vi "Advanced settings MAX.vi"(1 "Admin Path":string="C:\\Data Log\\Admin") -> (0 "output cluster":T1)   [LabVIEW 2014]
uses:
  <vilib>/Utility/file.llb/Read From Spreadsheet File (DBL).vi
panel:
  out "SMS Recipients":u32
  in  "SMS":bool
  in  "Mexa 7170":bool
  out "Boolean":bool
  in  "Leak Test":bool
  in  "OK Button":bool
  in  "Bottle":bool
  in  "Logging":bool
  in  "System":bool
  in  "Lambda":bool
  out "Tab Control":T2(tab)
  in  "Inlet TC":dbl=1.0 min=1.0 max=32.0
  in  "Bed TC":dbl=1.0 min=1.0 max=32.0
  in  "Cycle Length":dbl=500.0
  in  "Heat Load Control":bool
  in  "Purge Duration":dbl=30.0
  in  "Reference Temp":dbl=700.0
  in  "Target Heat Load":dbl
  in  "C Factor":dbl=21000.0
  in  "Directory":string="C:\\Data Log"
  in  "ETAS":bool
  in  "MKS":bool
  in  "Mexa 1":bool
  in  "Mexa 2":bool
  in  "Mexa 3":bool
  in  "Log Interval":dbl=4.0
  in  "Vehicle Name":string="V1"
  in  "Nicky":bool
  in  "Kurtis":bool
  in  "Andy":bool
  in  "Ryan":bool
  in  "Liam":bool
  in  "Matthew":bool
  in  "Calvin":bool
  in  "Text Alerts":bool
  in  "Lambda Control On/Off":bool
  in  "D":dbl min=0.0 max=100.0
  in  "I":dbl min=0.0 max=100.0
  in  "P":dbl min=0.0 max=100.0
  in  "Lambda Target":dbl min=0.0 max=100.0
  in  "O2 Concentration":dbl=100.0 min=0.0 max=100.0
  in  "Propane":bool
  in  "CO Concentration":dbl=100.0 min=0.0 max=100.0
  in  "HC Concentration":dbl=100.0 min=0.0 max=100.0
  in  "NOx Concentration":dbl=100.0 min=0.0 max=100.0
  in  "Air Bal":bool
  in  "N2":bool
  in  "Duration Leak Test":dbl min=0.0 max=100.0
  # "Advanced Settings"
  # "System Settings"
  # "s"
  # "hr"
  # "Advanced Settings"
  # "Data Log Settings"
  # "hr"
  # "Advanced Settings"
  # "SMS Alert Settings"
  # "SMS Recipients"
  # "Advanced Settings"
  # "Lambda Control Settings"
  # "Advanced Settings"
  # "Gas Settings"
  # "%"
  # "%"
  # "%"
  # "%"
  # "Advanced Settings"
  # "Leak Test Settings"
  # "s"
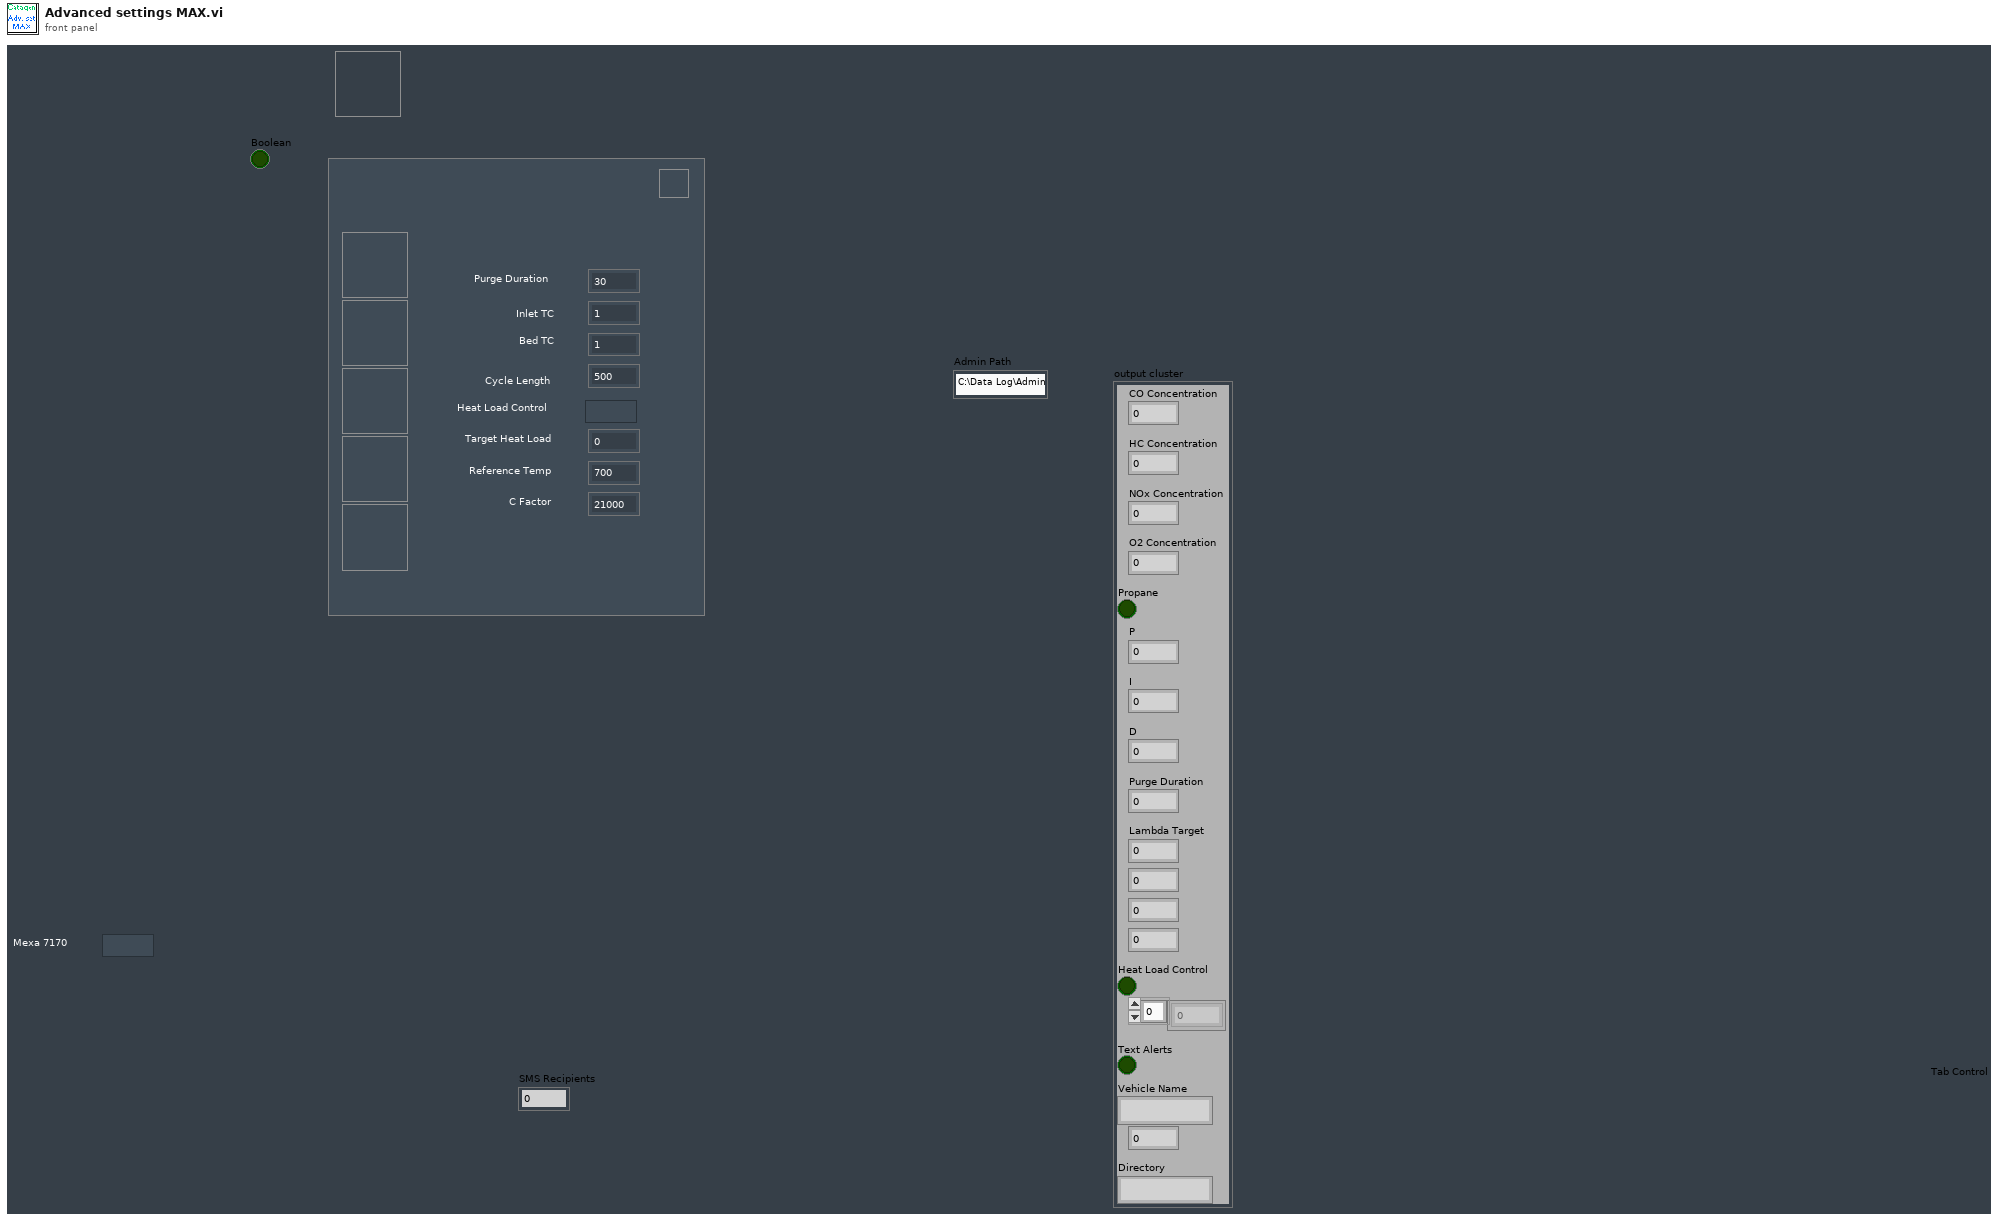
[diagram p1: front panel]
types:
  T1 = cluster{"CO Concentration":dbl, "HC Concentration":dbl, "NOx Concentration":dbl, "O2 Concentration":dbl, "Propane":bool, "P":dbl, "I":dbl, "D":dbl, "Purge Duration":dbl, "Lambda Target":dbl, dbl, u32, dbl, "Heat Load Control":bool, dbl[], "Text Alerts":bool, "Vehicle Name":string, u32, "Directory":string}
  T2 = enum32{"System ", "Logging", "SMS", "Lambda", "Bottle", "Leak Test"}
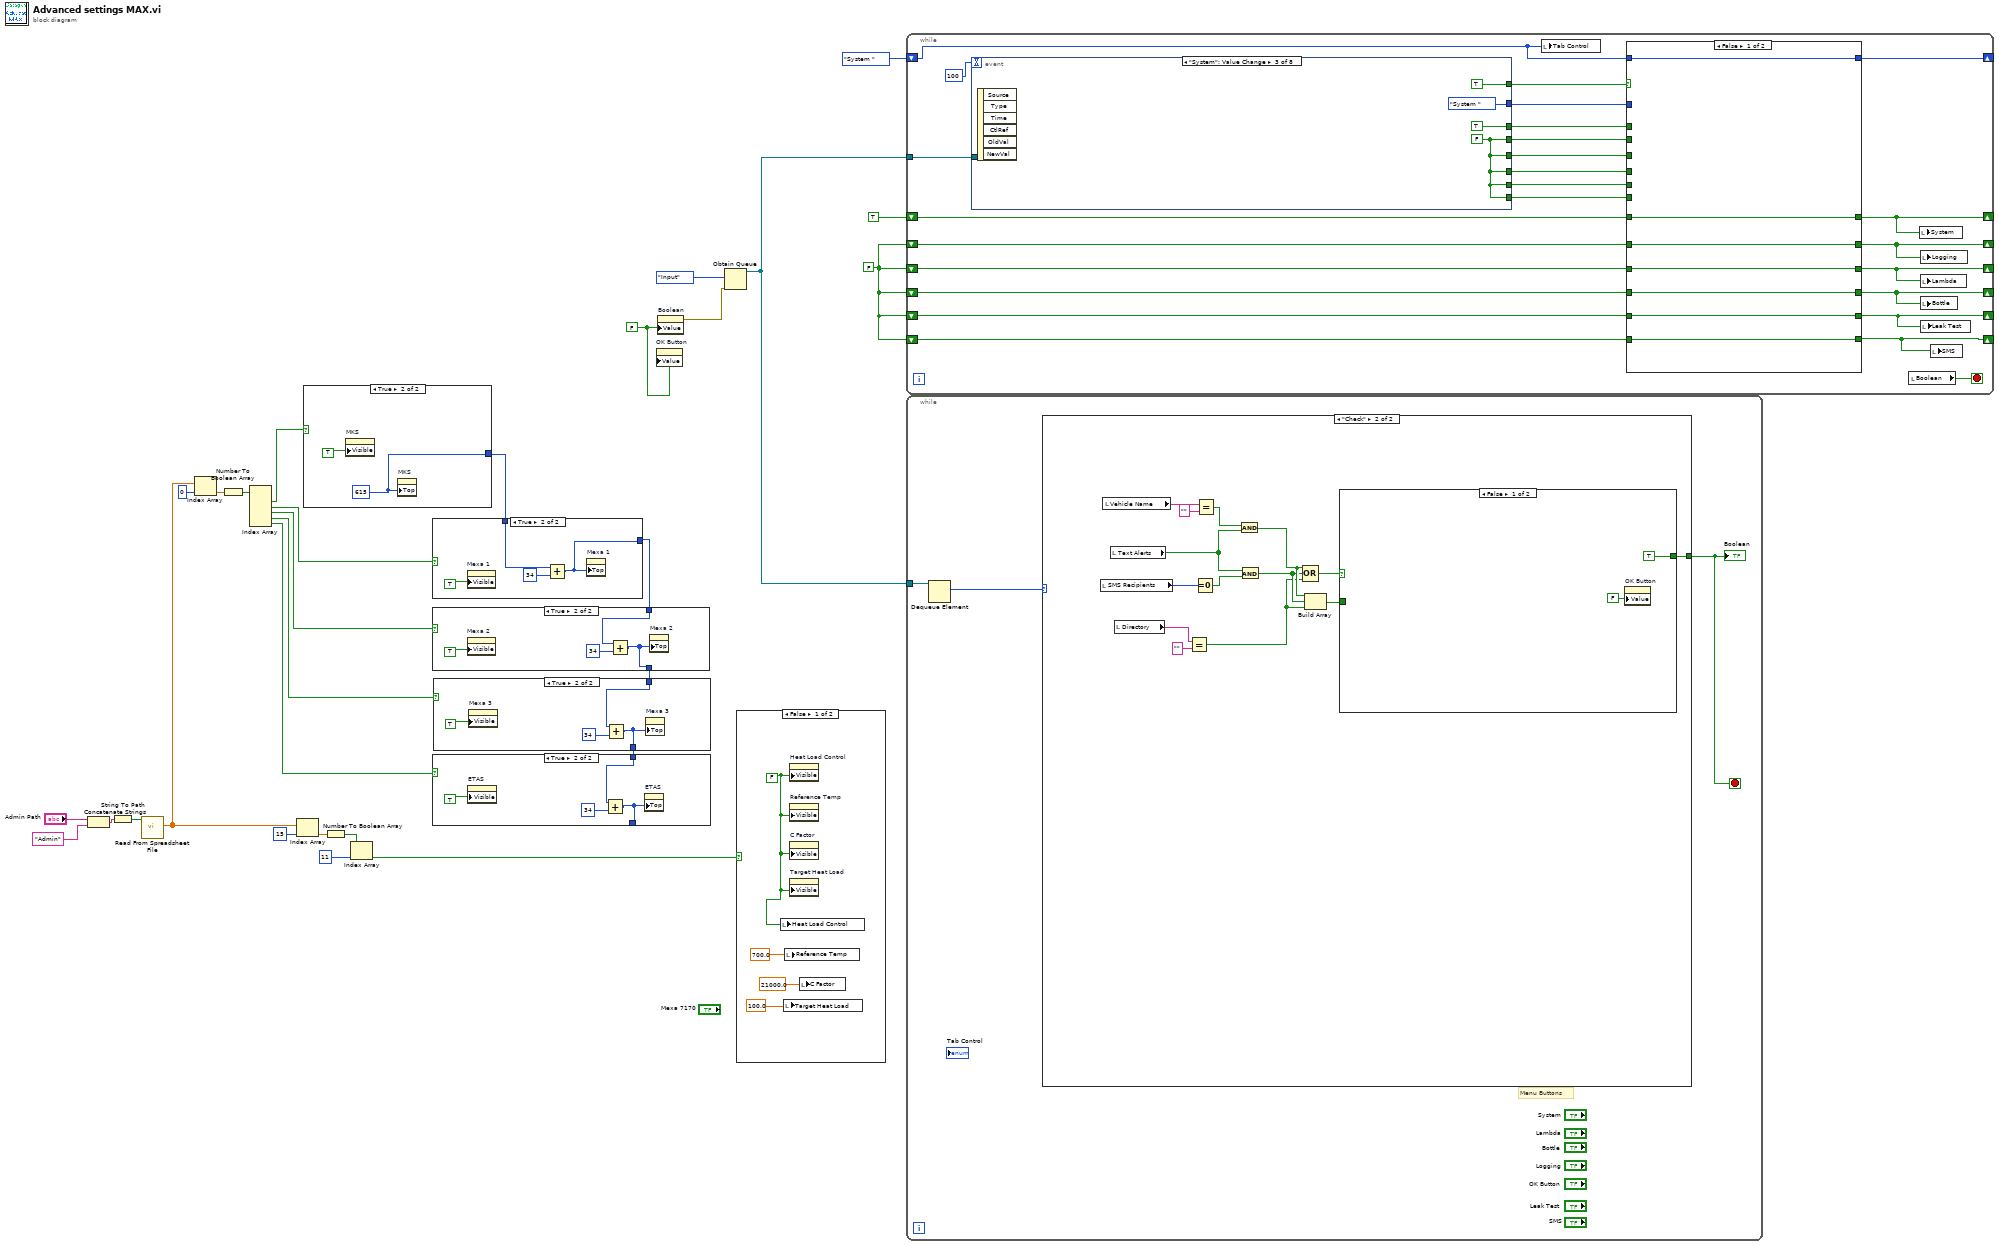
[diagram p0: block diagram]
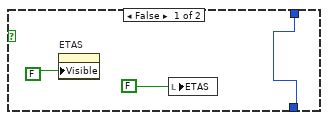
[diagram p2: hidden frame]
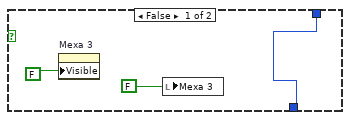
[diagram p3: hidden frame]
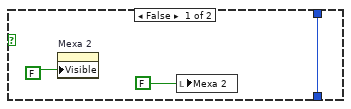
[diagram p4: hidden frame]
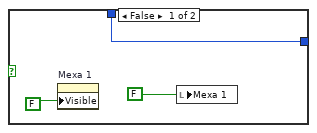
[diagram p5: hidden frame]
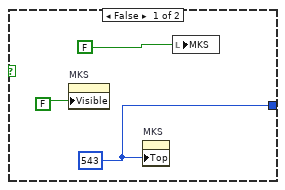
[diagram p6: hidden frame]
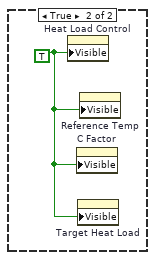
[diagram p7: hidden frame]
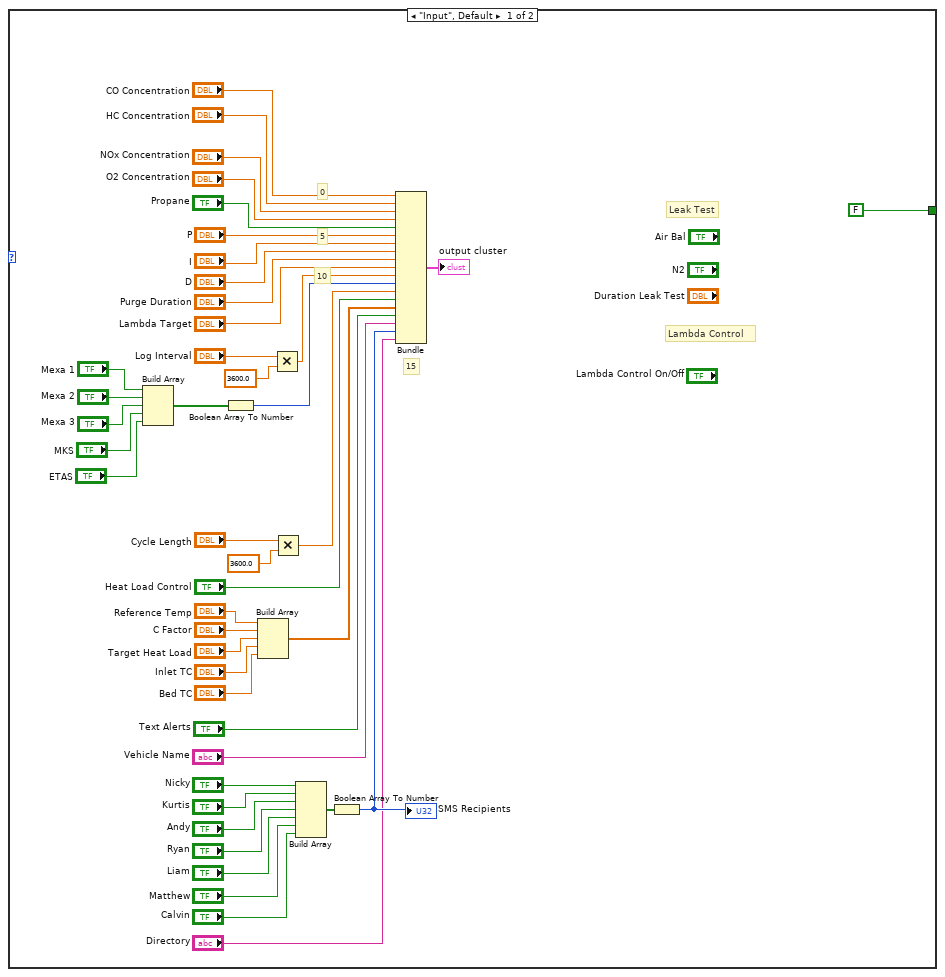
[diagram p8: hidden frame]
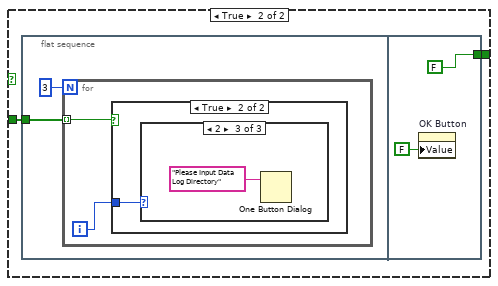
[diagram p9: hidden frame]
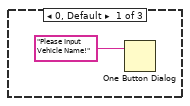
[diagram p11: hidden frame]
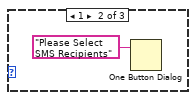
[diagram p12: hidden frame]
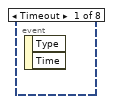
[diagram p14: hidden frame]
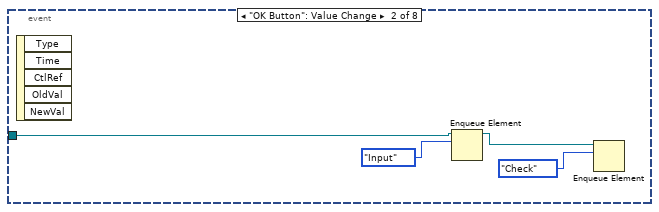
[diagram p15: hidden frame]
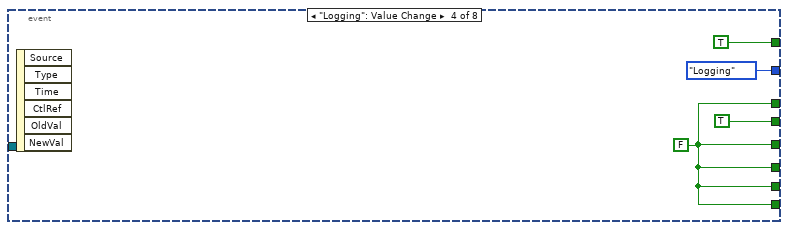
[diagram p16: hidden frame]
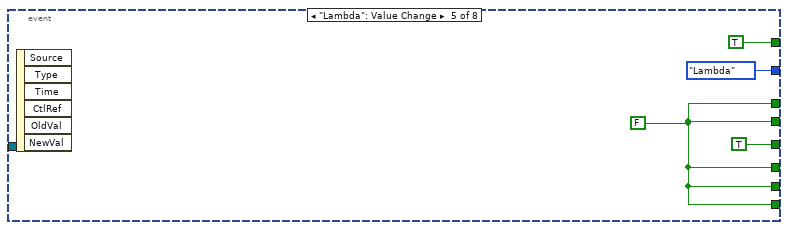
[diagram p17: hidden frame]
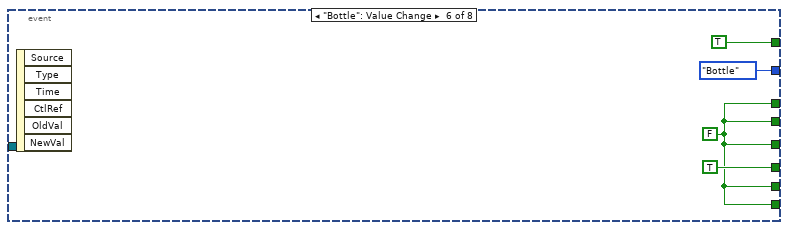
[diagram p18: hidden frame]
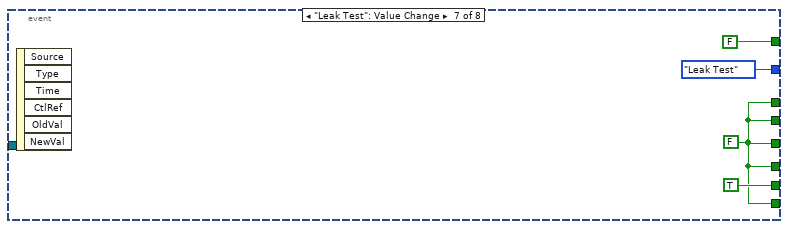
[diagram p19: hidden frame]
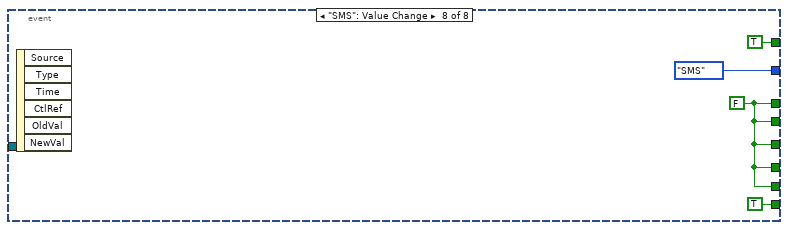
[diagram p20: hidden frame]
diagram:
  w26 = FALSE ("Boolean")
  w1 = FALSE ("s")
  n1 = Concatenate Strings("Admin Path", "Admin" ("string")) -> (w13:string)
  n2 = String To Path(string=w13) -> (path=w24:path)
  n3 = call-poly <vilib>:"Read From Spreadsheet File.vi"("file path (dialog if empty)"=w24) -> ("first row"=w11:dbl[])  [unwired: 6 in, 4 out]
  n4 = Index Array(array=w11, index=0) -> (element=w9:dbl)
  n5 = Number To Boolean Array(number=w9) -> (Boolean array=w8:bool[])
  n6 = Index Array(array=w8) -> (element #1=w7:bool, element #2=w6:bool, element #3=w5:bool, element #4=w4:bool, element #5=w3:bool)  [unwired: 5 in]
  n7 = Index Array(array=w11, index=15) -> (element=w23:dbl)
  n8 = case shown="True" w7 {
    tunnel: [w30 w33] -> w18
    frame False {
      w30 = 543 ("Position:Top")
      n9 = property on="MKS" class="Bool (strict)"("Visible"=FALSE) -> ()  [unwired: 2 in, 2 out]
      n10 = property on="MKS" class="Bool (strict)"("Top"=w30) -> ()  [unwired: 2 in, 2 out]
      n11 = local write "MKS"(FALSE ("Mexa One")) -> ()
    }
    frame True {
      w33 = 615 ("Position:Top")
      n12 = property on="MKS" class="Bool (strict)"("Visible"=TRUE) -> ()  [unwired: 2 in, 2 out]
      n13 = property on="MKS" class="Bool (strict)"("Top"=w33) -> ()  [unwired: 2 in, 2 out]
    }
  }
  n14 = Number To Boolean Array(number=w23) -> (Boolean array=w20:bool[])
  n15 = Index Array(array=w20, index=11) -> (element=w19:bool)
  n16 = case shown="True" w6 {
    tunnel: w18 -> [w35 w39]
    tunnel: [w35 w38] -> w17
    frame False {
      n17 = property on="Mexa 1" class="Bool (strict)"("Visible"=FALSE) -> ()  [unwired: 2 in, 2 out]
      n18 = local write "Mexa 1"(FALSE ("Mexa 584a")) -> ()
    }
    frame True {
      n19 = property on="Mexa 1" class="Bool (strict)"("Visible"=TRUE) -> ()  [unwired: 2 in, 2 out]
      n20 = Add(x=w39, y=34) -> (x+y=w38:i32)
      n21 = property on="Mexa 1" class="Bool (strict)"("Top"=w38) -> ()  [unwired: 2 in, 2 out]
    }
  }
  n22 = case shown="True" w5 {
    tunnel: w17 -> [w42 w46]
    tunnel: [w42 w45] -> w16
    frame False {
      n23 = property on="Mexa 2" class="Bool (strict)"("Visible"=FALSE) -> ()  [unwired: 2 in, 2 out]
      n24 = local write "Mexa 2"(FALSE ("Mexa 584b")) -> ()
    }
    frame True {
      n25 = property on="Mexa 2" class="Bool (strict)"("Visible"=TRUE) -> ()  [unwired: 2 in, 2 out]
      n26 = Add(x=w46, y=34) -> (x+y=w45:i32)
      n27 = property on="Mexa 2" class="Bool (strict)"("Top"=w45) -> ()  [unwired: 2 in, 2 out]
    }
  }
  n28 = case shown="True" w4 {
    tunnel: w16 -> [w49 w53]
    tunnel: [w49 w52] -> w12
    frame False {
      n29 = property on="Mexa 3" class="Bool (strict)"("Visible"=FALSE) -> ()  [unwired: 2 in, 2 out]
      n30 = local write "Mexa 3"(FALSE ("Mexa 7170")) -> ()
    }
    frame True {
      n31 = property on="Mexa 3" class="Bool (strict)"("Visible"=TRUE) -> ()  [unwired: 2 in, 2 out]
      n32 = Add(x=w53, y=34) -> (x+y=w52:i32)
      n33 = property on="Mexa 3" class="Bool (strict)"("Top"=w52) -> ()  [unwired: 2 in, 2 out]
    }
  }
  n34 = case shown="True" w3 {
    tunnel: w12 -> [w56 w60]
    tunnel: [w56 w59] -> _
    frame False {
      n35 = property on="ETAS" class="Bool (strict)"("Visible"=FALSE) -> ()  [unwired: 2 in, 2 out]
      n36 = local write "ETAS"(FALSE ("Mexa 7170")) -> ()
    }
    frame True {
      n37 = property on="ETAS" class="Bool (strict)"("Visible"=TRUE) -> ()  [unwired: 2 in, 2 out]
      n38 = Add(x=w60, y=34) -> (x+y=w59:i32)
      n39 = property on="ETAS" class="Bool (strict)"("Top"=w59) -> ()  [unwired: 2 in, 2 out]
    }
  }
  n40 = property on="OK Button" class="Bool (strict)"("Value"=w26) -> ()  [unwired: 2 in, 2 out]
  n41 = property on="Boolean" class="Bool (strict)"("Value"=w26) -> (error out=w25:errorcluster)  [unwired: 2 in, 1 out]
  n42 = Obtain Queue(element data type=enum16{"Input", "Check"}."Input", error in (no error)=w25) -> (queue out=w28:refnum<queue>)  [unwired: 3 in, 2 out]
  n43 = case shown="False" w19 {
    frame False {
      w66 = FALSE ("Visible")
      n44 = local write "Heat Load Control"(w66) -> ()
      n45 = local write "Target Heat Load"(100.0 ("Target Heat Load")) -> ()
      n46 = local write "Reference Temp"(700.0 ("Reference Temp")) -> ()
      n47 = property on="Heat Load Control" class="Bool (strict)"("Visible"=w66) -> ()  [unwired: 2 in, 2 out]
      n48 = property on="Reference Temp" class="DigNum (strict)"("Visible"=w66) -> ()  [unwired: 2 in, 2 out]
      n49 = property on="C Factor" class="DigNum (strict)"("Visible"=w66) -> ()  [unwired: 2 in, 2 out]
      n50 = property on="Target Heat Load" class="DigNum (strict)"("Visible"=w66) -> ()  [unwired: 2 in, 2 out]
      n51 = local write "C Factor"(21000.0 ("C Factor")) -> ()
    }
    frame True {
      w67 = TRUE ("Visible")
      n52 = property on="Heat Load Control" class="Bool (strict)"("Visible"=w67) -> ()  [unwired: 2 in, 2 out]
      n53 = property on="C Factor" class="DigNum (strict)"("Visible"=w67) -> ()  [unwired: 2 in, 2 out]
      n54 = property on="Target Heat Load" class="DigNum (strict)"("Visible"=w67) -> ()  [unwired: 2 in, 2 out]
      n55 = property on="Reference Temp" class="DigNum (strict)"("Visible"=w67) -> ()  [unwired: 2 in, 2 out]
    }
  }
  n56 = while {
    tunnel: w28 -> [w91]
    shift-right: [w89] -> _
    shift-left: T2."System " ("Tab Control") -> [w72]
    shift-right: [w87] -> _
    shift-left: w1 -> [w88]
    shift-right: [w82] -> _
    shift-left: TRUE ("s") -> [w81]
    shift-right: [w80] -> _
    shift-left: w1 -> [w79]
    shift-right: [w78] -> _
    shift-left: w1 -> [w77]
    shift-right: [w73] -> _
    shift-left: w1 -> [w74]
    shift-right: [w68] -> _
    shift-left: w1 -> [w71]
    stop <- w75 stop-if-true
    n57 = event shown="[2] \"System\": Value Change" {
      selector: _ -> [_ _ _ _ _ _ _ _]
      dyn-events: _ -> [_ _ _ _ _ _ _ _]
      timeout: 100 -> [_ _ _ _ _ _ _ _]
      tunnel: w91 -> [_ w110 _ _ _ _ _ _]
      tunnel: [_ _ TRUE ("s") TRUE ("s") TRUE ("s") TRUE ("s") FALSE ("s") TRUE ("s")] -> w90
      tunnel: [_ _ w111 w115 TRUE ("s") w124 w128 w131] -> w85
      tunnel: [_ _ TRUE ("s") w115 w120 w124 w128 w131] -> w83
      tunnel: [_ _ w111 TRUE ("s") w120 w124 w128 w131] -> w84
      tunnel: [_ _ w111 w115 w120 TRUE ("s") w128 w131] -> w86
      tunnel: [_ _ w111 w115 w120 w124 TRUE ("s") w131] -> w76
      tunnel: [_ _ T2."System " ("Tab Control") T2."Logging" ("Tab Control") T2."Lambda" ("Tab Control") T2."Bottle" ("Tab Control") T2."Leak Test" ("Tab Control") T2."SMS" ("Tab Control")] -> w70
      tunnel: [_ _ w111 w115 w120 w124 w128 TRUE ("s")] -> w69
      event Timeout {
        n58 = event-data() -> ()  [unwired: 1 in, 2 out]
      }
      event "OK Button": Value Change {
        n59 = event-data() -> ()  [unwired: 1 in, 5 out]
        n60 = Enqueue Element(queue=w110, element=enum16{"Input", "Check"}."Input") -> (queue out=w107:refnum<queue>)  [unwired: 2 in, 2 out]
        n61 = Enqueue Element(queue=w107, element=enum16{"Input", "Check"}."Check") -> ()  [unwired: 2 in, 3 out]
      }
      event "System": Value Change {
        w111 = FALSE ("s")
        n62 = event-data() -> ()  [unwired: 1 in, 6 out]
      }
      event "Logging": Value Change {
        w115 = FALSE ("s")
        n63 = event-data() -> ()  [unwired: 1 in, 6 out]
      }
      event "Lambda": Value Change {
        w120 = FALSE ("s")
        n64 = event-data() -> ()  [unwired: 1 in, 6 out]
      }
      event "Bottle": Value Change {
        w124 = FALSE ("s")
        n65 = event-data() -> ()  [unwired: 1 in, 6 out]
      }
      event "Leak Test": Value Change {
        w128 = FALSE ("s")
        n66 = event-data() -> ()  [unwired: 1 in, 6 out]
      }
      event "SMS": Value Change {
        w131 = FALSE ("s")
        n67 = event-data() -> ()  [unwired: 1 in, 6 out]
      }
    }
    n68 = local write "Tab Control"(w72) -> ()
    n69 = case shown="False" w90 {
      tunnel: w70 -> [_ w106]
      tunnel: [w99 w106] -> w89
      tunnel: w72 -> [w99 _]
      tunnel: w88 -> [w98 _]
      tunnel: [w98 w105] -> w87
      tunnel: w86 -> [_ w105]
      tunnel: w85 -> [_ w104]
      tunnel: w84 -> [_ w103]
      tunnel: w83 -> [_ w102]
      tunnel: [w97 w104] -> w78
      tunnel: [w96 w103] -> w80
      tunnel: [w95 w102] -> w82
      tunnel: w81 -> [w95 _]
      tunnel: w79 -> [w96 _]
      tunnel: w77 -> [w97 _]
      tunnel: w76 -> [_ w101]
      tunnel: w74 -> [w94 _]
      tunnel: [w94 w101] -> w73
      tunnel: w71 -> [w93 _]
      tunnel: [w93 w100] -> w68
      tunnel: w69 -> [_ w100]
      frame False {
      }
      frame True {
      }
    }
    n70 = local read "Boolean"() -> (w75:bool)
    n71 = local write "System"(w82) -> ()
    n72 = local write "Logging"(w80) -> ()
    n73 = local write "Lambda"(w78) -> ()
    n74 = local write "Bottle"(w87) -> ()
    n75 = local write "Leak Test"(w73) -> ()
    n76 = local write "SMS"(w68) -> ()
  }
  n77 = while {
    tunnel: w28 -> [w137]
    stop <- w135 stop-if-true
    # "Menu Buttons"
    n78 = Dequeue Element(queue=w137) -> (element=w136:enum16{"Input", "Check"})  [unwired: 2 in, 3 out]
    n79 = case shown="\"Check\"" w136 {
      tunnel: [FALSE w186] -> w135
      frame "Input", Default {
        # "Lambda Control"
        # "Leak Test"
        # "15"
        # "10"
        # "5"
        # "0"
        n80 = Build Array("Mexa 1", "Mexa 2", "Mexa 3", "MKS", "ETAS") -> (w162:bool[])
        n81 = Boolean Array To Number(Boolean array=w162) -> (number=w161:u32)
        n82 = Build Array("Reference Temp", "C Factor", "Target Heat Load", "Inlet TC", "Bed TC") -> (w178:dbl[])
        n83 = Multiply(x="Log Interval", y=3600.0) -> (x*y=w180:dbl)
        n84 = Multiply(x="Cycle Length", y=3600.0) -> (x*y=w179:dbl)
        n85 = Build Array("Nicky", "Kurtis", "Andy", "Ryan", "Liam", "Matthew", "Calvin") -> (w142:bool[])
        n86 = Boolean Array To Number(Boolean array=w142) -> (number=w141:u32)
        "SMS Recipients" <- w141
        n87 = Bundle("CO Concentration"="CO Concentration", "HC Concentration"="HC Concentration", "NOx Concentration"="NOx Concentration", "O2 Concentration"="O2 Concentration", "Propane"="Propane", "P"="P", "I"="I", "D"="D", "Purge Duration"="Purge Duration", "Lambda Target"="Lambda Target", w180, w161, w179, "Heat Load Control"="Heat Load Control", w178, "Text Alerts"="Text Alerts", "Vehicle Name"="Vehicle Name", w141, "Directory"="Directory") -> (→"output cluster":T1)  [unwired: 1 in]
      }
      frame "Check" {
        n88 = local read "SMS Recipients"() -> (w194:u32)
        n89 = local read "Vehicle Name"() -> (w192:string)
        n90 = local read "Text Alerts"() -> (w193:bool)
        n91 = local read "Directory"() -> (w189:string)
        n92 = Equal?(x=w189, y="") -> (x = y?=w183:bool)
        n93 = Equal To 0?(x=w194) -> (x = 0?=w195:bool)
        n94 = Equal?(x=w192, y="") -> (x = y?=w190:bool)
        n95 = And(x=w190, y=w193) -> (x .and. y?=w185:bool)
        n96 = And(x=w193, y=w195) -> (x .and. y?=w184:bool)
        n97 = Compound Arithmetic op=OR(w185, w184, w183) -> (w187:bool)
        n98 = Build Array(w185, w184, w183) -> (w182:bool[])
        n99 = case shown="False" w187 {
          tunnel: [TRUE w198] -> w186
          tunnel: w182 -> [_ w199]
          frame False {
            n100 = property on="OK Button" class="Bool (strict)"("Value"=FALSE ("OK Button")) -> ()  [unwired: 2 in, 2 out]
          }
          frame True {
            n101 = flat-sequence {
              tunnel: w199 -> [w200]
              tunnel: [FALSE ("OK Button")] -> w198
              frame #0 {
                n102 = for {
                  N: 3 -> [_]
                  tunnel: w200 -> [w203] mode=indexing
                  i -> [w202]
                  n103 = case shown="True" w203 {
                    tunnel: w202 -> [_ w204]
                    frame False {
                    }
                    frame True {
                      n104 = case shown="2" w204 {
                        frame 0, Default {
                          n105 = One Button Dialog(message="Please Input Vehicle Name!") -> ()  [unwired: 1 in, 1 out]
                        }
                        frame 1 {
                          n106 = One Button Dialog(message="Please Select SMS Recipients") -> ()  [unwired: 1 in, 1 out]
                        }
                        frame 2 {
                          n107 = One Button Dialog(message="Please Input Data Log Directory") -> ()  [unwired: 1 in, 1 out]
                        }
                      }
                    }
                  }
                }
              }
              frame #1 {
                n108 = property on="OK Button" class="Bool (strict)"("Value"=FALSE ("OK Button")) -> ()  [unwired: 2 in, 2 out]
              }
            }
          }
        }
      }
    }
    "Boolean" <- w135
  }
